vi "Pending Stock Design.vi"(8 "error in (no error)":errorcluster) -> (0 "error out":errorcluster, 1 "Pending":i16, 2 "Need a design":bool, 3 "DesignRequest":T1, 4 "Successful Checkout":bool, 5 "Mathcad version":i32)   [LabVIEW 2012]
uses:
  Design Request.ctl
  Variable cluster.ctl
  Design Server.lvlib
panel:
  out "Method Index":i32
  out "Stock Design Index":i32
  out "Method Name":string
  out "Request File Name":string
  out "Needed":bool[][](array[boolean])
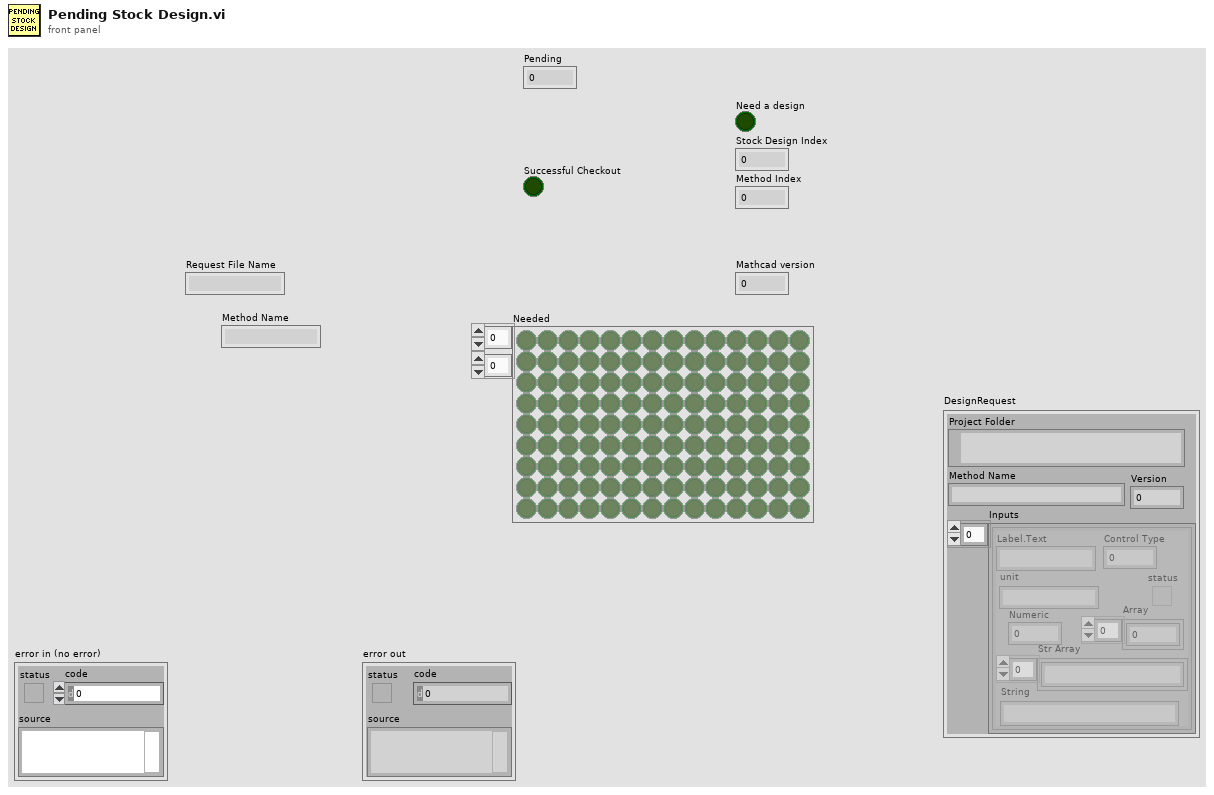
[diagram p1: front panel]
types:
  T1 = typedef "Design Server.lvlib/Design Request.ctl" = cluster{"Project Folder":path, "Method Name":string, "Inputs":T2, "Version":i32}
  T2 = typedef "Design Server.lvlib/Variable cluster.ctl" = cluster{"Label.Text":string, "Control Type":u32, "Numeric":dbl, "Array":dbl[], "status":bool, "Str Array":string[], "String":string, "unit":string}[]
  T3 = typedef "Method.ctl" = cluster{"Title":string, "About":string, "Input Parameters":cluster{"Description":string, "Name":string, "Min":string, "Max":string, "Default":string, "Units":string, "Increment":string, "Stock designs":string[]}[], "AutoCAD drawings":cluster{"File Name":string, "AC Variables":string[]}[], "Stock file names":string[], "Publish files":string[], "Display images":string[]}
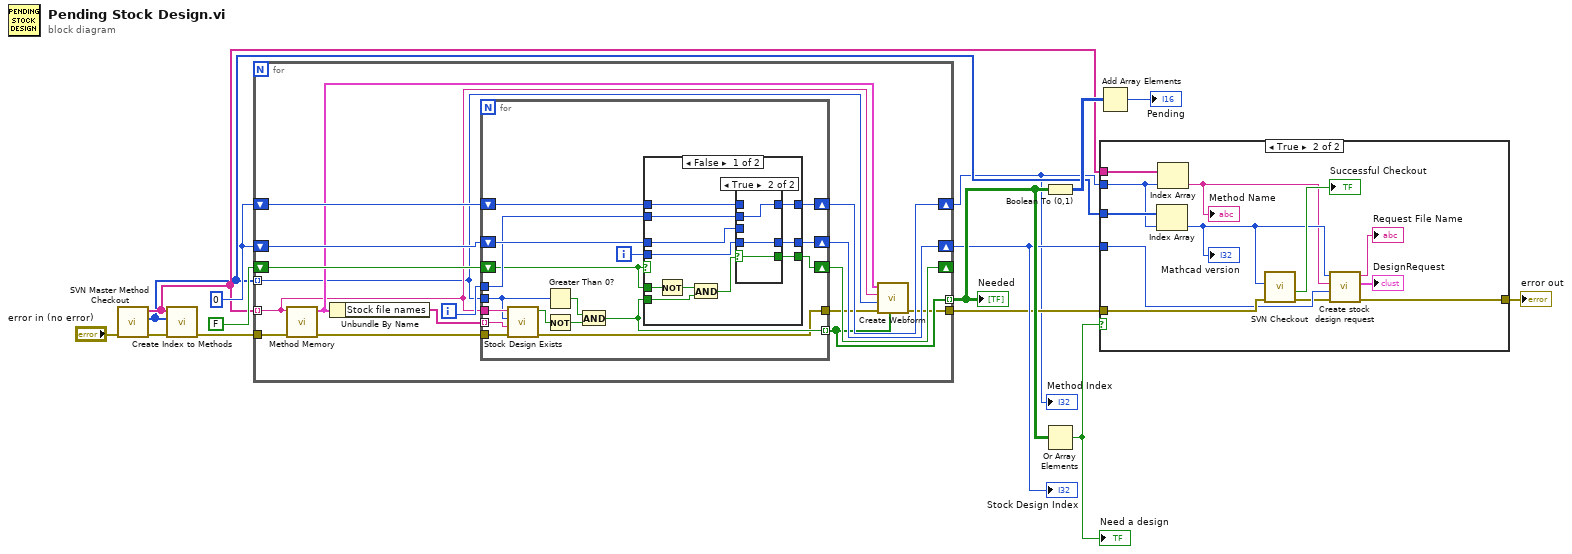
[diagram p0: block diagram]
diagram:
  w14 = 0
  n1 = call "SVN Master Method Checkout.vi"("error in (no error)"="error in (no error)") -> ("error out"=w3:errorcluster, "versions"=w4:i32[], "Method Names"=w5:string[])  [unwired: 5 in, 3 out]
  n2 = call "Create Index to Methods.vi"("error in"=w3, "versions"=w4, "Method Names"=w5) -> ("error out"=w2:errorcluster)  [unwired: 8 in]
  n3 = for {
    tunnel: w5 -> [w19] mode=indexing
    tunnel: w4 -> [w18] mode=indexing
    tunnel: [w21] -> w13 mode=indexing
    shift-right: [w31] -> _
    shift-left: FALSE -> [w30]
    shift-right: [w28] -> w10
    shift-left: w14 -> [w29]
    shift-right: [w27] -> w1
    shift-left: w14 -> [w26]
    tunnel: [w16] -> w8
    tunnel: w2 -> [w23]
    i -> [w25]
    n4 = call "Method Memory.vi"("error in"=w23, "Method Name"=w19) -> ("error out"=w24:errorcluster, "Method Out"=w20:T3)  [unwired: 7 in, 1 out]
    n5 = Unbundle By Name(w20) -> ("Stock file names"=w22:string[])
    n6 = for {
      tunnel: w19 -> [w48]
      tunnel: w18 -> [w46]
      tunnel: w22 -> [w47] mode=indexing
      tunnel: [w42] -> w21 mode=indexing
      shift-right: [w35] -> w31
      shift-left: w30 -> [w34]
      shift-right: [w41] -> w28
      shift-left: w29 -> [w39]
      shift-right: [w38] -> w27
      shift-left: w26 -> [w36]
      tunnel: w25 -> [w37]
      tunnel: w24 -> [w33]
      tunnel: [w32] -> w17
      i -> [w40]
      n7 = call "Stock Design Exists.vi"("error in (no error)"=w33, "Request File Name"=w47, "Revision"=w46, "Method"=w48) -> ("error out"=w32:errorcluster, "file or folder exists?"=w45:bool)  [unwired: 6 in]
      n8 = Greater Than 0?(x=w46) -> (x > 0?=w43:bool)
      n9 = Not(x=w45) -> (.not. x?=w44:bool)
      n10 = And(x=w43, y=w44) -> (x .and. y?=w42:bool)
      n11 = case shown="False" w34 {
        tunnel: w34 -> [w59 w68]
        tunnel: w42 -> [w57 _]
        tunnel: [w55 w67] -> w41
        tunnel: w40 -> [w54 _]
        tunnel: w39 -> [w53 w67]
        tunnel: [w52 w66] -> w38
        tunnel: w37 -> [w51 _]
        tunnel: w36 -> [w50 w66]
        tunnel: [w49 w68] -> w35
        frame False {
          n12 = Not(x=w59) -> (.not. x?=w58:bool)
          n13 = And(x=w58, y=w57) -> (x .and. y?=w56:bool)
          n14 = case shown="True" w56 {
            selector: w56 -> [w62 w65]
            tunnel: [w62 w65] -> w49
            tunnel: [w61 w64] -> w55
            tunnel: w54 -> [_ w64]
            tunnel: w53 -> [w61 _]
            tunnel: [w60 w63] -> w52
            tunnel: w51 -> [_ w63]
            tunnel: w50 -> [w60 _]
            frame False {
            }
            frame True {
            }
          }
        }
        frame True {
        }
      }
    }
    n15 = call "Create Webform.vi"("Under Construction"=w21, "error in (no error)"=w17, "Mathcad version"=w18, "Method Name"=w19, "Method"=w20) -> ("error out"=w16:errorcluster)  [unwired: 5 in, 1 out]
  }
  "Needed" <- w13
  "Stock Design Index" <- w10
  "Method Index" <- w1
  n16 = Boolean To (0,1)(Boolean=w13) -> (0, 1=w12:i16[][])
  n17 = Or Array Elements(Boolean array=w13) -> (logical OR=w9:bool)
  "Need a design" <- w9
  n18 = Add Array Elements(numeric array=w12) -> (sum=→"Pending":i16)
  n19 = case shown="True" w9 {
    tunnel: w4 -> [_ w81]
    tunnel: w1 -> [_ w80]
    tunnel: w10 -> [_ w74]
    tunnel: w5 -> [_ w77]
    tunnel: w8 -> [w69 w79]
    tunnel: [w69 w70] -> w7
    frame False {
    }
    frame True {
      n20 = Index Array(array=w81, index=w80) -> (element=w76:i32)
      "Mathcad version" <- w76
      n21 = Index Array(array=w77, index=w80) -> (element=w75:string)
      "Method Name" <- w75
      n22 = call "SVN Checkout.vi"("error in (no error)"=w79, "ADT version"=w76) -> ("error out"=w73:errorcluster, "Successful Checkout"=→"Successful Checkout":bool)  [unwired: 6 in, 2 out]
      n23 = call "Create stock design request.vi"("error in"=w73, "Stock Design Index"=w74, "Method Name"=w75, "Mathcad version"=w76) -> ("error out"=w70:errorcluster, "DesignRequest"=→"DesignRequest":T1, "Request File Name"=→"Request File Name":string)  [unwired: 5 in]
    }
  }
  "error out" <- w7
